vi "ARRAY II.vi"() -> ()   [LabVIEW 2022 SP3]
panel:
  out "max index(es)":i32
  out "min value":i32
  out "min index(es)":i32
  out "max value":i32
  out "deleted portion":i32[](array[numeric])
  out "array w/ subset deleted":i32[](array[numeric])
  out "output array 2":i32[][](array[numeric])
  out "output array":i32[](array[numeric])
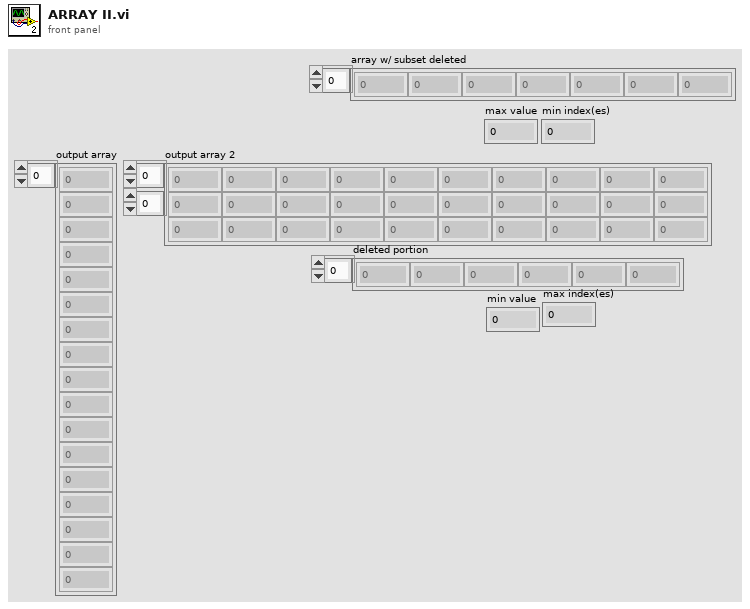
[diagram p1: front panel]
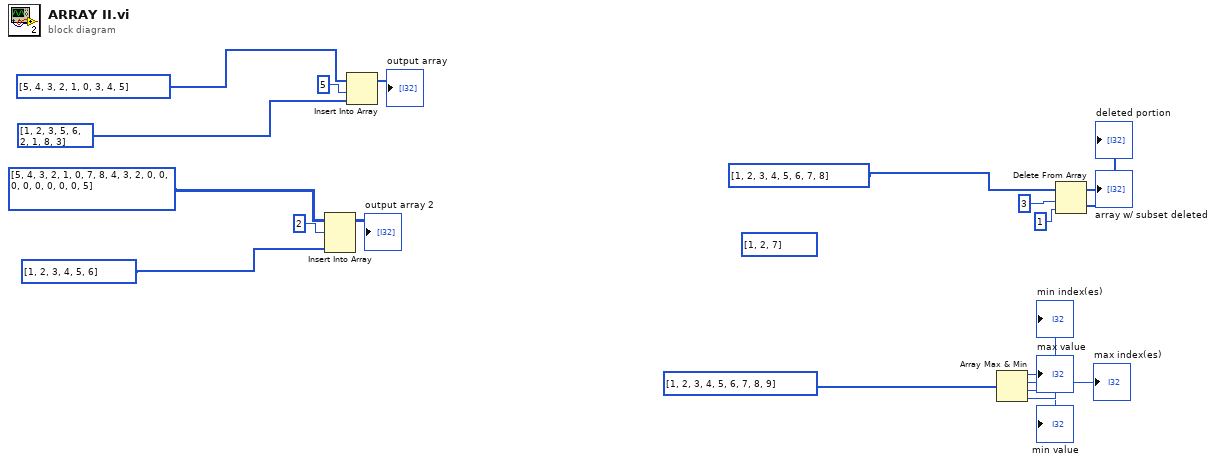
[diagram p0: block diagram]
diagram:
  (unwired) i32[] [1, 2, 7]
  n1 = Insert Into Array(array=i32[][] [[5, 4, 3, 2, 1, 0, 7, 8, 4, 3], [2, 0, 0, 0, 0, 0, 0, 0, 0, 5]], index (row)=2 ("index"), new element=i32[] [1, 2, 3, 4, 5, 6]) -> (→"output array 2":i32[][])  [unwired: 1 in]
  n2 = Insert Into Array(array=i32[] [5, 4, 3, 2, 1, 0, 3, 4, 5], index=5, new element=i32[] [1, 2, 3, 5, 6, 2, 1, 8, 3]) -> (→"output array":i32[])
  n3 = Array Max & Min(array=i32[] [1, 2, 3, 4, 5, 6, 7, 8, 9]) -> (max value=→"max value":i32, max index (indices)=→"max index(es)":i32, min value=→"min value":i32, min index (indices)=→"min index(es)":i32)
  n4 = Delete From Array(array=i32[] [1, 2, 3, 4, 5, 6, 7, 8], length=3, index=1) -> (deleted portion=→"deleted portion":i32[], array with subset deleted=→"array w/ subset deleted":i32[])
